vi "SVFA Compensate Phase for Reference Frequencies.vi"   [LabVIEW 2017]
doc: "Use this VI to enable vector averaging of complex spectra even when the frequencies of interest do not have constant phase incidence in the measurement window (analysis block)."
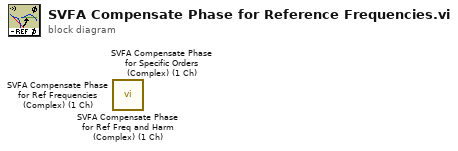
[diagram p0: block diagram]
diagram:
  n1 = call <vilib>:"SVFA Compensate Phase for Ref Freq and Harm (Complex) (1 Ch).vi"() -> ()  [unwired: 18 in, 2 out]
  n2 = call <vilib>:"SVFA Compensate Phase for Specific Orders (Complex) (1 Ch).vi"() -> ()  [unwired: 18 in, 2 out]
  n3 = call <vilib>:"SVFA Compensate Phase for Ref Frequencies (Complex) (1 Ch).vi"() -> ()  [unwired: 18 in, 2 out]
